vi "Handle GU Arrange List Menu Event.vi"(6 "Top VI":refnum<vi>, 8 "error in":errorcluster, 9 "Coords":T1, 10 "ItemTag":string, 11 "CtlRef":refnum<vi>) -> (0 "error out":errorcluster, 3 "Next Case":string[](array[string]))   [LabVIEW 2020, in "GUCalibration2.lvlib"]
uses:
  GUCalibration2.lvlib
  <vilib>/Utility/miscctls.llb/LVPoint32TypeDef.ctl
  <vilib>/Utility/miscctls.llb/LVRowAndColumnTypeDef.ctl
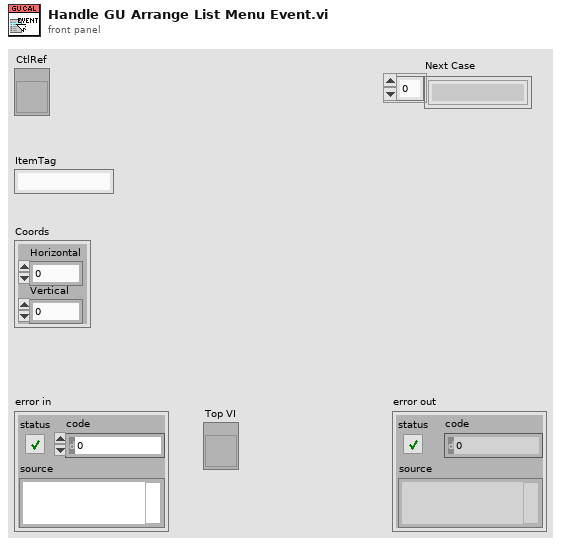
[diagram p1: front panel]
types:
  T1 = typedef "LVPoint32TypeDef.ctl" = cluster{"Horizontal":i32, "Vertical":i32}
  T2 = typedef "LVRowAndColumnTypeDef.ctl" = cluster{"Row":i32, "Column":i32}
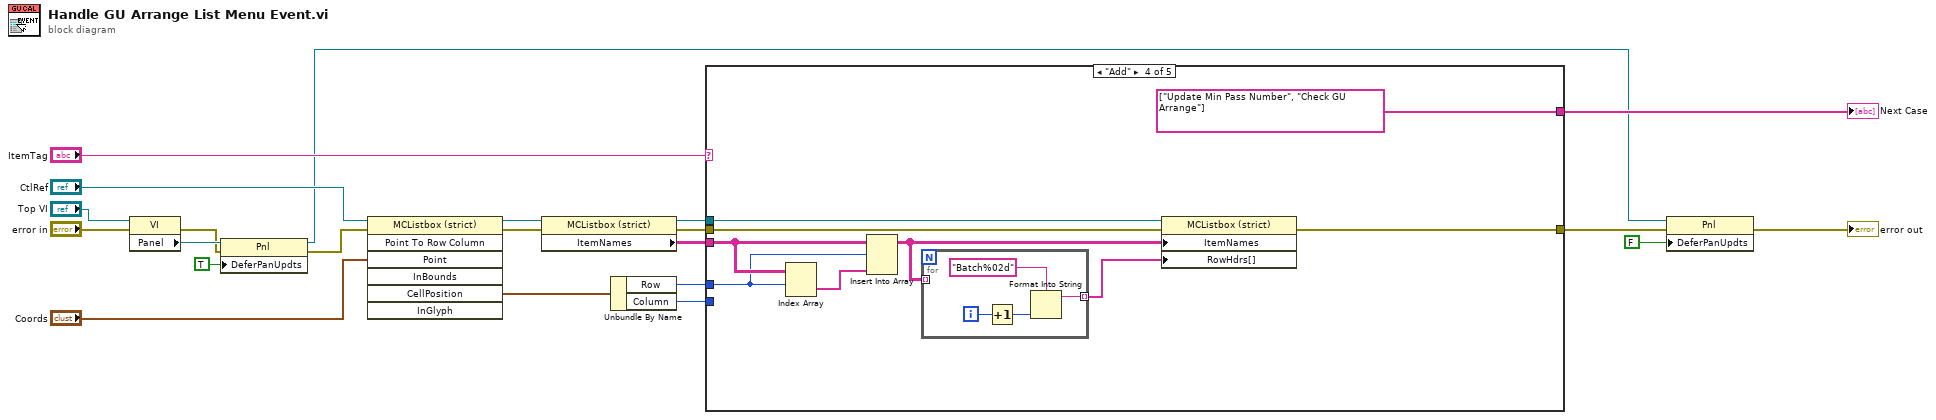
[diagram p0: block diagram]
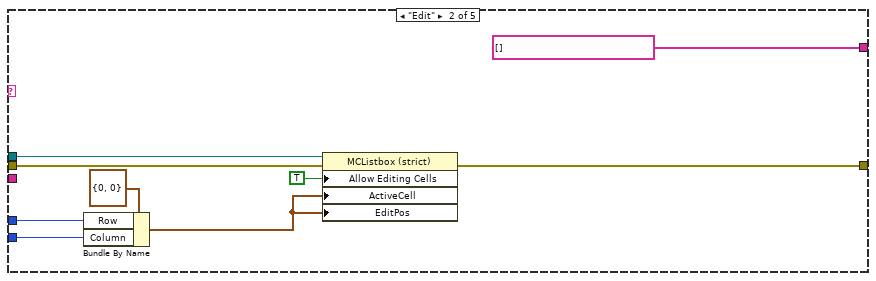
[diagram p3: hidden frame]
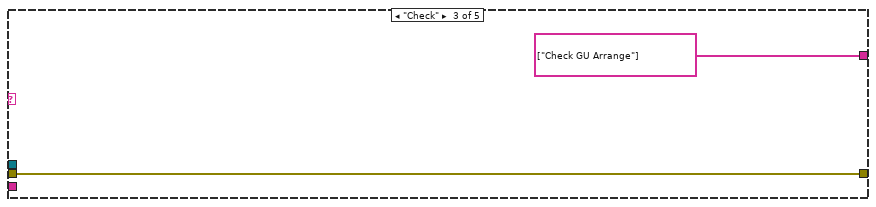
[diagram p4: hidden frame]
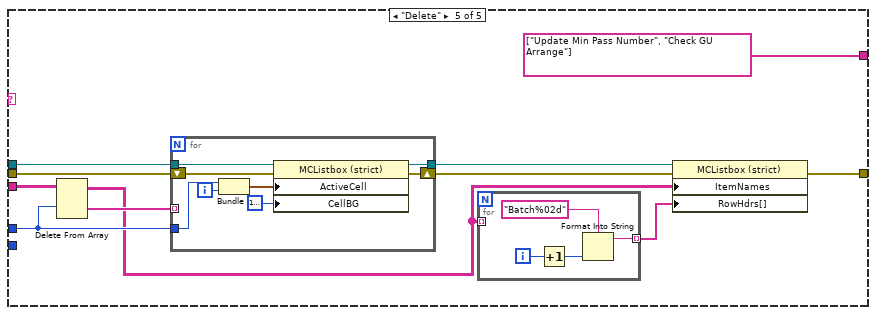
[diagram p5: hidden frame]
diagram:
  n1 = property class="VI"(reference="Top VI", error in="error in") -> (error out=w8:errorcluster, "Panel"=w10:refnum<vi>)  [unwired: 1 out]
  n2 = property class="Pnl"(reference=w10, error in=w8, "DeferPanUpdts"=TRUE ("Defer Panel Updates")) -> (reference out=w1:refnum<vi>, error out=w6:errorcluster)
  n3 = invoke class="MCListbox (strict)" method="Point To Row Column"(reference="CtlRef", error in=w6, "Point"="Coords") -> (reference out=w16:refnum<vi>, error out=w15:errorcluster, "CellPosition"=w14:T2)  [unwired: 4 in, 4 out]
  n4 = property class="MCListbox (strict)"(reference=w16, error in=w15) -> (reference out=w19:refnum<vi>, error out=w21:errorcluster, "ItemNames"=w20:string[][])
  n5 = Unbundle By Name(w14) -> ("Row"=w13:i32, "Column"=w12:i32)
  n6 = case shown="\"Add\"" "ItemTag" {
    tunnel: w21 -> [w23 w31 w34 w42 w55]
    tunnel: w20 -> [_ _ _ w41 w58]
    tunnel: w19 -> [_ w32 _ w43 w56]
    tunnel: w13 -> [_ w29 _ w39 w53]
    tunnel: w12 -> [_ w28 _ _ _]
    tunnel: [w23 w27 w34 w37 w50] -> w3
    tunnel: [_ string[] [] string[] ["Check GU Arrange"] string[] ["Update Min Pass Number", "Check GU Arrange"] string[] ["Update Min Pass Number", "Check GU Arrange"]] -> w11
    frame "False", Default {
    }
    frame "Edit" {
      n7 = Bundle By Name(cluster=T2 {"Row"=0, "Column"=0} ("Edit Position"), "Row"=w29, "Column"=w28) -> (w26:T2)
      n8 = property class="MCListbox (strict)"(reference=w32, error in=w31, "Allow Editing Cells"=TRUE, "ActiveCell"=w26, "EditPos"=w26) -> (error out=w27:errorcluster)  [unwired: 1 out]
    }
    frame "Check" {
    }
    frame "Add" {
      n9 = Index Array(array=w41, index (row)=w39) -> (element=w40:string[])  [unwired: 1 in]
      n10 = Insert Into Array(array=w41, index (row)=w39, new element=w40) -> (w38:string[][])  [unwired: 1 in]
      n11 = for {
        tunnel: w38 -> [_] mode=indexing
        tunnel: [w44] -> w36 mode=indexing
        i -> [w46]
        n12 = Increment(x=w46) -> (x+1=w47:i32)
        n13 = Format Into String(format string="Batch%02d", w47) -> (resulting string=w44:string)  [unwired: 2 in, 1 out]
      }
      n14 = property class="MCListbox (strict)"(reference=w43, error in=w42, "ItemNames"=w38, "RowHdrs[]"=w36) -> (error out=w37:errorcluster)  [unwired: 1 out]
    }
    frame "Delete" {
      n15 = Delete From Array(array=w58, index (row)=w53) -> (deleted portion=w54:string[], array with subset deleted=w51:string[][])  [unwired: 2 in]
      n16 = for {
        tunnel: w56 -> [w65]
        shift-right: [w63] -> w52
        shift-left: w55 -> [w66]
        tunnel: w54 -> [_] mode=indexing
        tunnel: w53 -> [w62]
        tunnel: [w59] -> w49
        i -> [w61]
        n17 = Bundle("Row"=w62, w61) -> (w60:cluster{"Row":i32, i32})  [unwired: 1 in]
        n18 = property class="MCListbox (strict)"(reference=w65, error in=w66, "ActiveCell"=w60, "CellBG"=u32 16777226) -> (reference out=w59:refnum<vi>, error out=w63:errorcluster)
      }
      n19 = for {
        tunnel: w51 -> [_] mode=indexing
        tunnel: [w67] -> w57 mode=indexing
        i -> [w69]
        n20 = Increment(x=w69) -> (x+1=w70:i32)
        n21 = Format Into String(format string="Batch%02d", w70) -> (resulting string=w67:string)  [unwired: 2 in, 1 out]
      }
      n22 = property class="MCListbox (strict)"(reference=w49, error in=w52, "ItemNames"=w51, "RowHdrs[]"=w57) -> (error out=w50:errorcluster)  [unwired: 1 out]
    }
  }
  "Next Case" <- w11
  n23 = property class="Pnl"(reference=w1, error in=w3, "DeferPanUpdts"=FALSE ("Defer Panel Updates")) -> (error out=→"error out":errorcluster)  [unwired: 1 out]
